vi "p41 bordesff.vi"() -> ()   [LabVIEW 2017]
panel:
  in  "Slide":dbl(slide) scale=0.0..255.0
  in  "path to BMP file":path
  out "new picture":picture
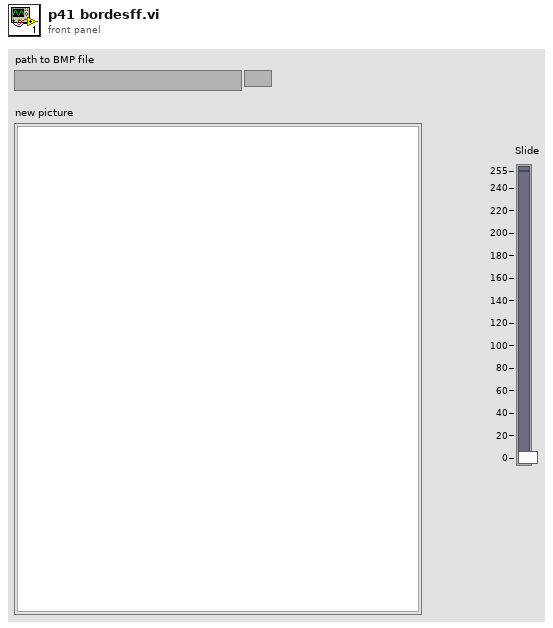
[diagram p1: front panel]
types:
  T1 = typedef "imagedata.ctl" = cluster{"image type":i32, "image depth":i32, "image":u8[], "mask":u8[], "colors":u32[], "Rectangle":cluster{"left":i16, "top":i16, "right":i16, "bottom":i16}}
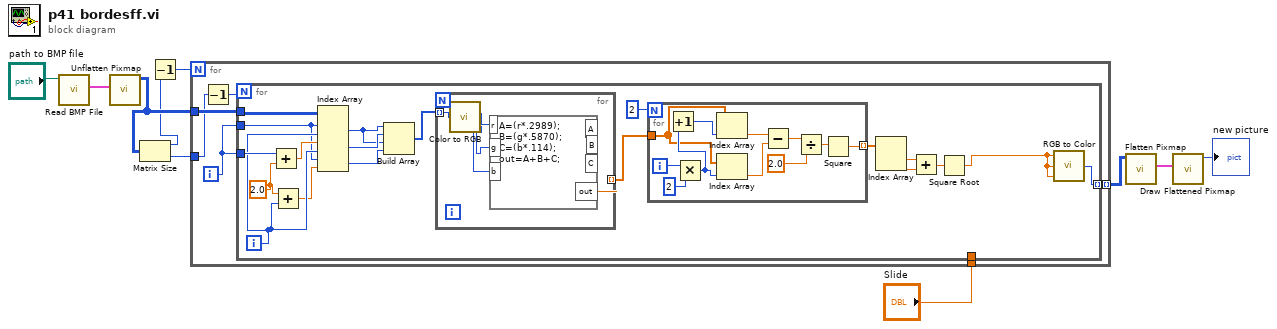
[diagram p0: block diagram]
diagram:
  n1 = call <vilib>:"Read BMP File.vi"("path to BMP file"="path to BMP file") -> ("image data"=w10:T1)  [unwired: 8 in, 2 out]
  n2 = call <vilib>:"Unflatten Pixmap.vi"("image data"=w10) -> ("24-bit pixmap"=w9:u32[][])  [unwired: 4 in, 6 out]
  n3 = Matrix Size(0:w9) -> (1:w8:i32, 2:w6:i32)
  n4 = Decrement(x=w8) -> (x-1=w7:i32)
  n5 = for {
    N: w7 -> [_]
    tunnel: w9 -> [w16]
    tunnel: w6 -> [w14]
    tunnel: [w12] -> w5 mode=indexing
    tunnel: "Slide" -> [w11]
    i -> [w13]
    n6 = Decrement(x=w14) -> (x-1=w15:i32)
    n7 = for {
      N: w15 -> [_]
      tunnel: w16 -> [w35]
      tunnel: w13 -> [w19]
      tunnel: w13 -> [w34]
      tunnel: [w22] -> w12 mode=indexing
      tunnel: w11 -> [_]
      i -> [w29]
      w30 = 2.0 ("y")
      n8 = Add(x=w34, y=w30) -> (x+y=w33:dbl)
      n9 = Add(x=w30, y=w29) -> (x+y=w18:dbl)
      n10 = Index Array(array=w35, index (row) #1=w19, index (col) #1=w29, index (row) #2=w33, index (col) #2=w29, index (row) #3=w19, index (col) #3=w18) -> (element #1=w21:u32, element #2=w32:u32, element #3=w20:u32)
      n11 = Build Array(w21, w32, w21, w20) -> (w31:u32[])
      n12 = for {
        tunnel: w31 -> [w48] mode=indexing
        tunnel: [w47] -> w27 mode=indexing
        n13 = call <vilib>:"Color to RGB.vi"("Color"=w48) -> ("R"=w51:u8, "G"=w50:u8, "B"=w49:u8)  [unwired: 1 out]
        n14 = formula code="A=(r*.2989);\nB=(g*.5870);\nC=(b*.114);\nout=A+B+C;"("r"=w51, "g"=w50, "b"=w49) -> ("out"=w47:dbl)  [unwired: 3 out]
      }
      n15 = for {
        N: 2 -> [_]
        tunnel: w27 -> [w41]
        tunnel: [w36] -> w26 mode=indexing
        i -> [w44]
        n16 = Multiply(x=w44, y=2) -> (x*y=w42:i32)
        n17 = Increment(x=w42) -> (x+1=w45:i32)
        n18 = Index Array(array=w41, index=w45) -> (element=w46:dbl)
        n19 = Index Array(array=w41, index=w42) -> (element=w40:dbl)
        n20 = Subtract(x=w46, y=w40) -> (x-y=w39:dbl)
        n21 = Divide(x=w39, y=2.0) -> (x/y=w37:dbl)
        n22 = Square(x=w37) -> (x^2=w36:dbl)
      }
      n23 = Index Array(array=w26) -> (element #1=w25:dbl, element #2=w24:dbl)  [unwired: 2 in]
      n24 = Add(x=w25, y=w24) -> (x+y=w23:dbl)
      n25 = Square Root(x=w23) -> (sqrt(x)=w17:dbl)
      n26 = call <vilib>:"RGB to Color.vi"("B"=w17, "G"=w17, "R"=w17) -> ("Color"=w22:u32)
    }
  }
  n27 = call <vilib>:"Flatten Pixmap.vi"("24-bit pixmap"=w5) -> ("image data"=w4:T1)  [unwired: 10 in]
  n28 = call <vilib>:"Draw Flattened Pixmap.vi"("image data"=w4) -> ("new picture"=→"new picture":picture)  [unwired: 8 in]
